vi "FTW-STR-Split.vi"(5 "Delimited String":string, 7 "Delimiter":string=",") -> (6 "Array of Strings":string[](array[string]))   [LabVIEW 2013]
uses:
  <vilib>/regexp/Match Regular Expression.xnode
panel:
  # "Inputs"
  # "Outputs"
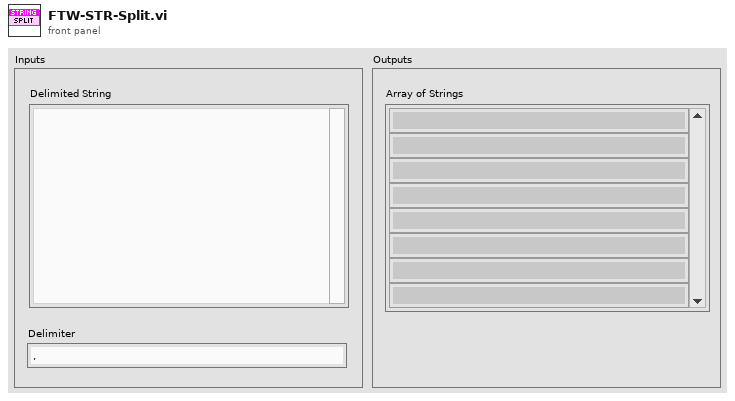
[diagram p1: front panel]
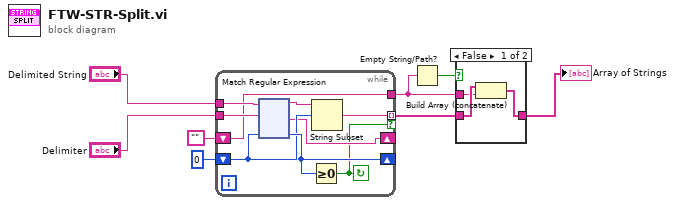
[diagram p0: block diagram]
diagram:
  n1 = while {
    tunnel: "Delimiter" -> [w17]
    tunnel: "Delimited String" -> [w16]
    shift-right: [w15] -> _
    shift-left: 0 ("offset past match") -> [w14]
    tunnel: [w12] -> w1 mode=indexing if=w9
    tunnel: [w10] -> w7
    shift-right: [w11] -> _
    shift-left: "" -> [w10]
    stop <- w9 continue-if-true
    n2 = xnode "Match Regular Expression"("input string"=w16, "regular expression"=w17, "offset (0)"=w14) -> ("before match"=w13:string, "after match"=w11:string, "offset past match"=w15:i32)  [unwired: 3 in, 2 out]
    n3 = Greater Or Equal To 0?(x=w15) -> (x >= 0?=w9:bool)
    n4 = String Subset(string=w13, offset (0)=w14) -> (substring=w12:string)  [unwired: 1 in]
  }
  n5 = Empty String/Path?(string/path=w7) -> (empty?=w6:bool)
  n6 = case shown="False" w6 {
    tunnel: w1 -> [w134 w135]
    tunnel: [w133 w135] -> w2
    tunnel: w7 -> [w132 _]
    frame False {
      n7 = Build Array (concatenate)(w134, w132) -> (w133:string[])
    }
    frame True {
    }
  }
  "Array of Strings" <- w2
